vi "writeTurret.vi"(8 "error in (no error)":errorcluster, 9 "Turret":T1, 10 "Pod Number":i32, 11 "Refnum in":T2) -> (0 "error out":errorcluster, 3 "Refnum out":T2)   [LabVIEW 2014]
uses:
  <vilib>/Utility/config.llb/Config Data RefNum.ctl
  <vilib>/Utility/config.llb/Write Key (Double).vi
  <vilib>/Utility/config.llb/Write Key (Boolean).vi
  <vilib>/Utility/config.llb/Write Key (String).vi
  <vilib>/Utility/config.llb/NI_LVConfig.lvlib
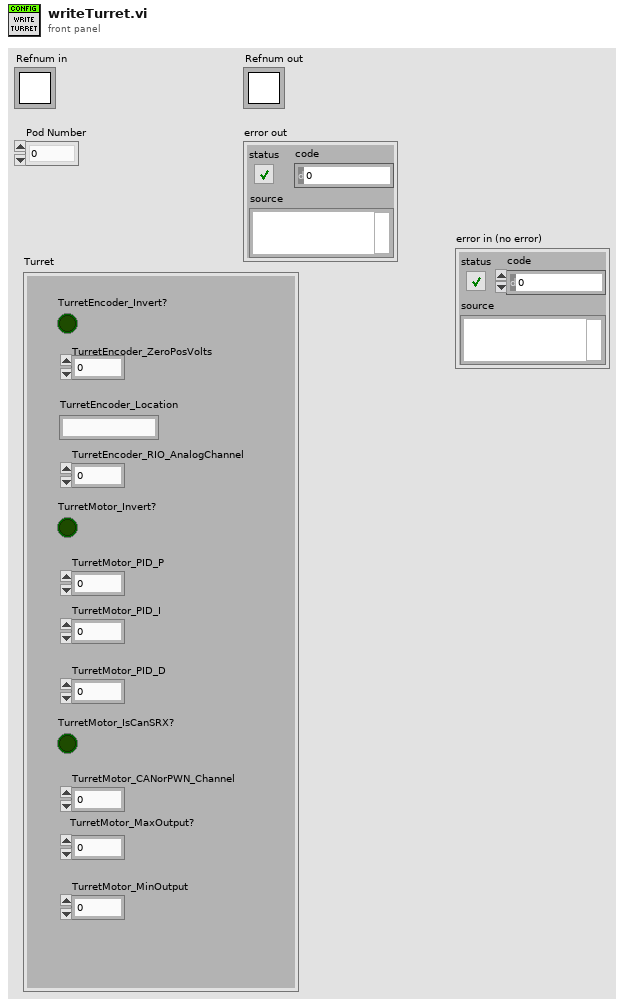
[diagram p1: front panel]
types:
  T1 = cluster{"TurretEncoder_Invert?":bool, "TurretEncoder_ZeroPosVolts":dbl, "TurretEncoder_Location":string, "TurretEncoder_RIO_AnalogChannel":dbl, "TurretMotor_Invert?":bool, "TurretMotor_PID_P":dbl, "TurretMotor_PID_I":dbl, "TurretMotor_PID_D":dbl, "TurretMotor_CANorPWN_Channel":dbl, "TurretMotor_IsCanSRX?":bool, "TurretMotor_MaxOutput?":dbl, "TurretMotor_MinOutput":dbl}
  T2 = typedef "NI_LVConfig.lvlib/Config Data RefNum.ctl" = refnum<k1>
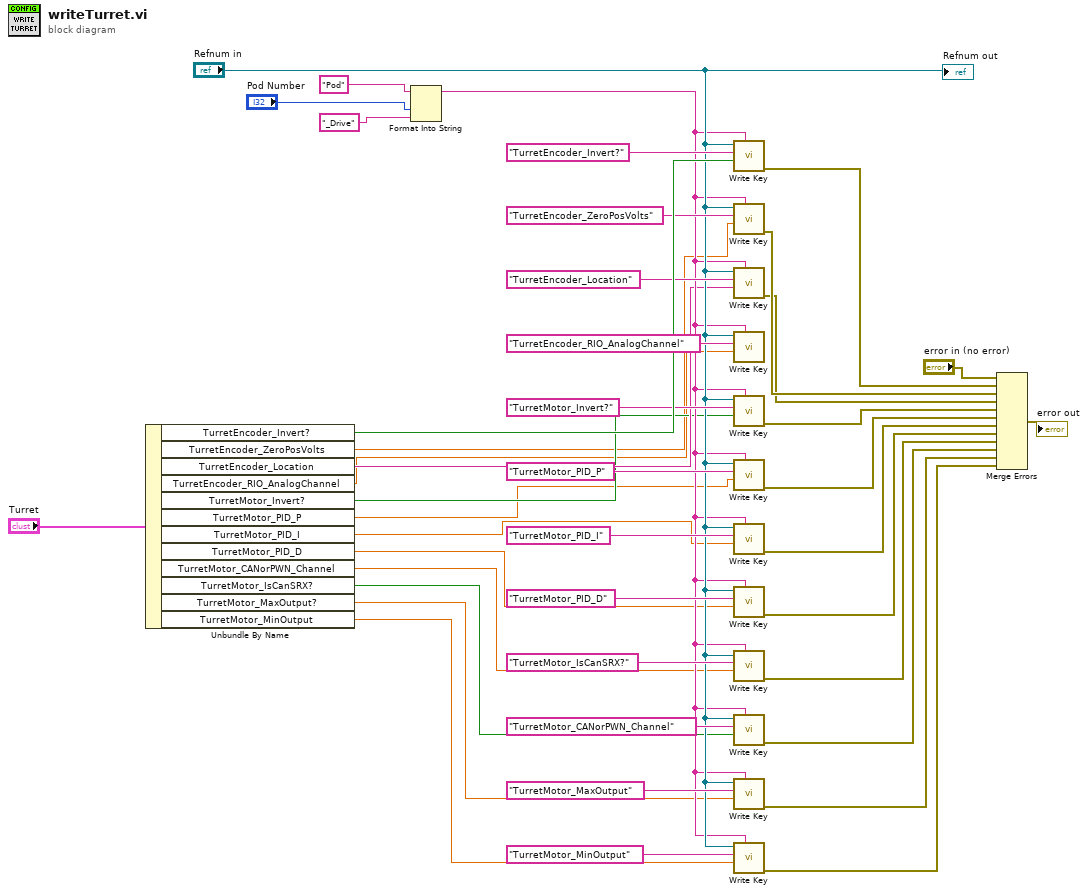
[diagram p0: block diagram]
diagram:
  n1 = Unbundle By Name("Turret") -> ("TurretEncoder_Invert?"=w43:bool, "TurretEncoder_ZeroPosVolts"=w15:dbl, "TurretEncoder_Location"=w25:string, "TurretEncoder_RIO_AnalogChannel"=w16:dbl, "TurretMotor_Invert?"=w24:bool, "TurretMotor_PID_P"=w23:dbl, "TurretMotor_PID_I"=w17:dbl, "TurretMotor_PID_D"=w18:dbl, "TurretMotor_CANorPWN_Channel"=w22:dbl, "TurretMotor_IsCanSRX?"=w19:bool, "TurretMotor_MaxOutput?"=w21:dbl, "TurretMotor_MinOutput"=w20:dbl)
  n2 = Format Into String(initial string="Pod", "Pod Number", "_Drive") -> (resulting string=w26:string)  [unwired: 2 in, 1 out]
  n3 = call-poly <vilib>:"Write Key.vi"("section"=w26, "value"=w43, "key"="TurretEncoder_Invert?", "refnum"="Refnum in") -> ("error out"=w14:errorcluster)  [unwired: 5 in, 2 out]
  n4 = call-poly <vilib>:"Write Key.vi"("section"=w26, "value"=w15, "key"="TurretEncoder_ZeroPosVolts", "refnum"="Refnum in") -> ("error out"=w13:errorcluster)  [unwired: 5 in, 2 out]
  n5 = call-poly <vilib>:"Write Key.vi"("section"=w26, "value"=w25, "key"="TurretEncoder_Location", "refnum"="Refnum in") -> ("error out"=w12:errorcluster)  [unwired: 5 in, 2 out]
  n6 = call-poly <vilib>:"Write Key.vi"("section"=w26, "value"=w16, "key"="TurretEncoder_RIO_AnalogChannel", "refnum"="Refnum in") -> ()  [unwired: 5 in, 3 out]
  n7 = call-poly <vilib>:"Write Key.vi"("section"=w26, "value"=w24, "key"="TurretMotor_Invert?", "refnum"="Refnum in") -> ("error out"=w11:errorcluster)  [unwired: 5 in, 2 out]
  n8 = call-poly <vilib>:"Write Key.vi"("section"=w26, "value"=w23, "key"="TurretMotor_PID_P", "refnum"="Refnum in") -> ("error out"=w10:errorcluster)  [unwired: 5 in, 2 out]
  n9 = call-poly <vilib>:"Write Key.vi"("section"=w26, "value"=w17, "key"="TurretMotor_PID_I", "refnum"="Refnum in") -> ("error out"=w9:errorcluster)  [unwired: 5 in, 2 out]
  n10 = call-poly <vilib>:"Write Key.vi"("section"=w26, "value"=w18, "key"="TurretMotor_PID_D", "refnum"="Refnum in") -> ("error out"=w8:errorcluster)  [unwired: 5 in, 2 out]
  n11 = call-poly <vilib>:"Write Key.vi"("section"=w26, "value"=w22, "key"="TurretMotor_IsCanSRX?", "refnum"="Refnum in") -> ("error out"=w7:errorcluster)  [unwired: 5 in, 2 out]
  n12 = call-poly <vilib>:"Write Key.vi"("section"=w26, "value"=w19, "key"="TurretMotor_CANorPWN_Channel", "refnum"="Refnum in") -> ("error out"=w6:errorcluster)  [unwired: 5 in, 2 out]
  n13 = call-poly <vilib>:"Write Key.vi"("section"=w26, "value"=w21, "key"="TurretMotor_MaxOutput", "refnum"="Refnum in") -> ("error out"=w5:errorcluster)  [unwired: 5 in, 2 out]
  n14 = call-poly <vilib>:"Write Key.vi"("section"=w26, "value"=w20, "key"="TurretMotor_MinOutput", "refnum"="Refnum in") -> ("error out"=w4:errorcluster)  [unwired: 5 in, 2 out]
  n15 = Merge Errors("error in (no error)", w14, w13, w12, w11, w10, w9, w8, w7, w6, w5, w4) -> (→"error out":errorcluster)
  "Refnum out" <- "Refnum in"
